vi "scale_to_zoom.vi"(8 "error in (no error)":errorcluster, 10 "offset found":i32[](array[numeric])=[0, 0], 11 "zoom":dbl) -> (0 "error out":errorcluster, 2 "offset found (scaled)":i32[](array[numeric]))   [LabVIEW 2010]
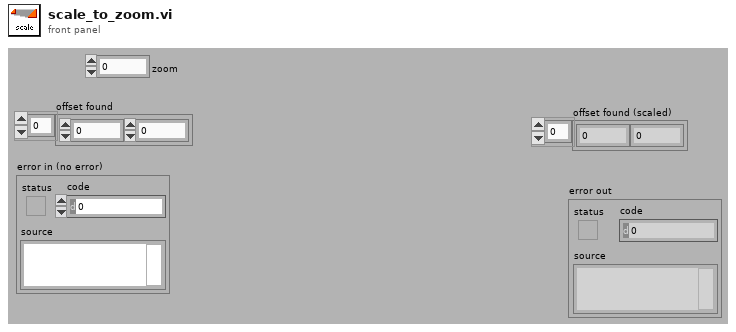
[diagram p1: front panel]
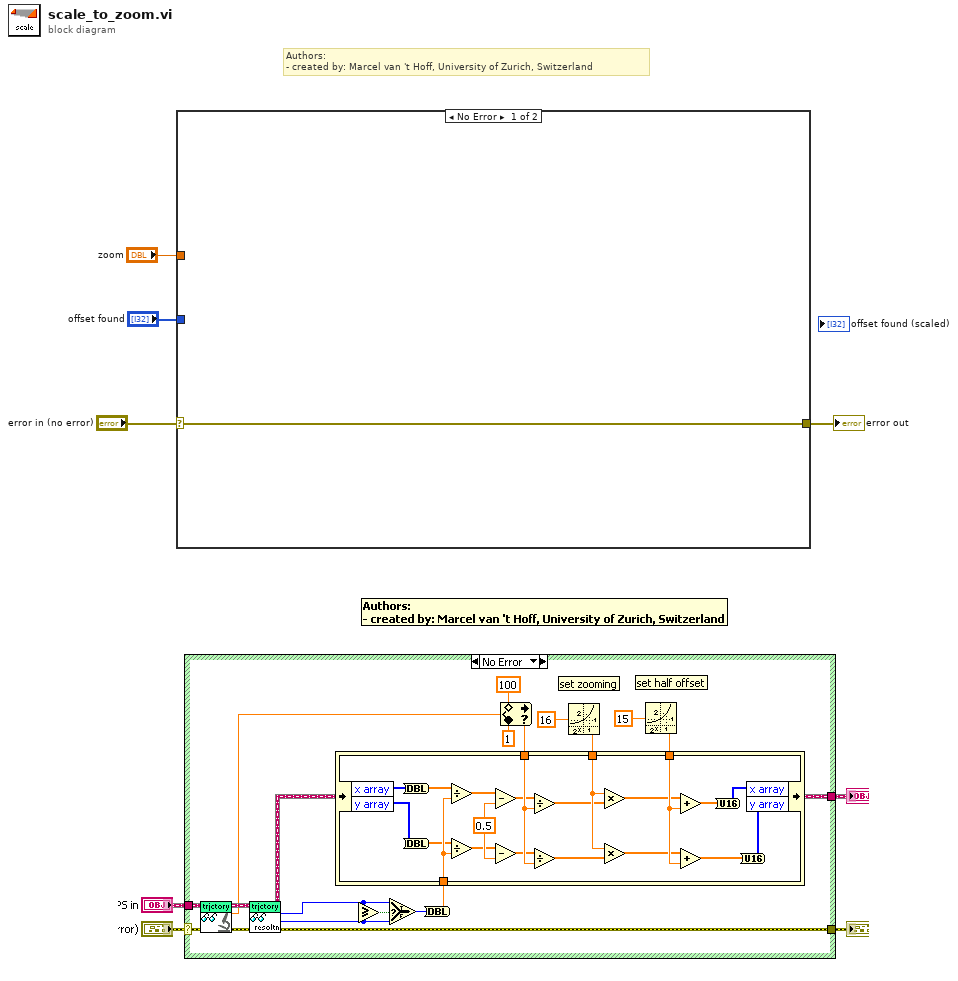
[diagram p0: block diagram]
diagram:
  # "Authors:\n- created by: Marcel van 't Hoff, University of Zurich, Switzerland"
  n1 = case shown="No Error" "error in (no error)" {
    selector: "error in (no error)" -> [w5 w6]
    tunnel: [w5 w6] -> w3
    tunnel: "offset found" -> [_ _]
    tunnel: "zoom" -> [_ _]
    frame No Error {
    }
    frame Error {
    }
  }
  "error out" <- w3
